vi "BonOMM-SAOMM.vi"() -> ()   [LabVIEW 2019] (continued)
                    n4150 = Concatenate Strings("FAPG.set -> (", w1579, ")") -> (w1577:string)
                    n4151 = call "TERMINAL.vi"("Indicateur Refnum"=w1582, "Terminal Refnum"=w1581, "Indicateur d'état"=w1577) -> ()
                    n4152 = call "SAOMM-SendSET.vi"("PRAMMS-COMM IN"=w1590, "Active Refnum"=w1588, "PrAMS-ACK"=w1587, "Signature"=w1584, "Error IN"=w1589, "MessageType"=w1586, "Active SET"="emtSetFPGACtrl", "Value (little endianed byte array)"=w1583) -> ("PRAMMS-COMM OUT"=w1592:refnum<visa-resource-name>, "Error OUT"=w1591:errorcluster)  [unwired: 4 in, 2 out]
                    n4153 = local write "PrAMS Error"(w1591) -> ()
                    n4154 = local write "PrAMS VRN"(w1592) -> ()
                  }
                  frame True {
                    n4155 = One Button Dialog(message="Impossible de modifier le FPGActrl pendant que la caméra fonctionne") -> ()  [unwired: 1 in, 1 out]
                  }
                }
              }
              event "Binning": Value Change {
                n4156 = event-data() -> ("OldVal"=w1598:u16, "NewVal"=w1597:u16)  [unwired: 1 in, 3 out]
                n4157 = local read "Integrating"() -> (w1595:bool)
                n4158 = local read "Servo"() -> (w1594:bool)
                n4159 = Or(x=w1595, y=w1594) -> (x .or. y?=w1596:bool)
                n4160 = case shown="Faux" w1596 {
                  tunnel: w1598 -> [w1610 _]
                  tunnel: w1597 -> [w1608 _]
                  frame False {
                    w1622 = "cam_Binning "
                    # "Passer dans une astrométrie ?"
                    n4161 = flat-sequence {
                      tunnel: [w1655] -> w1638
                      tunnel: [w1671] -> w1637
                      tunnel: w1638 -> [w1671]
                      tunnel: w1609 -> [w1663]
                      tunnel: w1607 -> [w1662]
                      tunnel: w1606 -> [w1661]
                      tunnel: [w1660] -> w1636
                      tunnel: [w1659] -> w1635
                      tunnel: [w1658] -> w1634
                      tunnel: w1637 -> [w1685]
                      tunnel: [w1682] -> w1605
                      tunnel: w1636 -> [w1682]
                      tunnel: w1635 -> [w1681]
                      tunnel: w1634 -> [w1676]
                      frame #0 {
                        n4162 = Tick Count (ms)() -> (millisecond timer value=w1655:u32)
                      }
                      frame #1 {
                        n4163 = control-ref of="PrAMS-ACK"() -> (w1656:refnum<vi>)
                        n4164 = local read "MessageType"() -> (w1665:cluster{string[], u32[]})
                        n4165 = control-ref of="PrAMS actif"() -> (w1657:refnum<vi>)
                        n4166 = local read "Signature"() -> (w1664:u32)
                        n4167 = local read "PrAMS VRN"() -> (w1670:refnum<visa-resource-name>)
                        n4168 = local read "PrAMS Error"() -> (w1669:errorcluster)
                        n4169 = call "SAOMM-BinningFixer.vi"("PRAMMS-COMM IN"=w1670, "Active Refnum"=w1657, "PrAMS-ACK"=w1656, "Signature"=w1664, "SendSET"=TRUE, "MessageType"=w1665, "Error IN"=w1669, "Binning"=w1663, "NAXIS"=w1661, "ROI Sizes"=w1662) -> ("PRAMMS-COMM OUT"=w1668:refnum<visa-resource-name>, "ScaleFactor"=w1660:dbl, "ROISizesOut"=w1659:T51, "ROIMinMax"=w1658:T52, "Error OUT"=w1667:errorcluster)  [unwired: 1 in]
                        n4170 = local write "PrAMS Error"(w1667) -> ()
                        n4171 = local write "PrAMS VRN"(w1668) -> ()
                      }
                      frame #2 {
                        n4172 = Tick Count (ms)() -> (millisecond timer value=w1684:u32)
                        n4173 = Subtract(x=w1684, y=w1685) -> (x-y=→"SetBinningTime":u32)
                        n4174 = Unbundle(w1681) -> ("ROIXOffset OUT"=w1680:u16, "ROIYOffset OUT"=w1679:u16, "ROIWidth OUT"=w1678:u16, "ROIHeight OUT"=w1677:u16)
                        n4175 = Unbundle(w1676) -> ("ROIXMin"=→"ROIXMin":u16, "ROIYXMax"=→"ROIXMax":u16, "ROIYMin"=→"ROIYMin":u16, "ROIYMax"=→"ROIYMax":u16)
                        n4176 = local write "ROIXOffset"(w1680) -> ()
                        n4177 = local write "ROIYOffset"(w1679) -> ()
                        n4178 = local write "ROIWidth"(w1678) -> ()
                        n4179 = local write "ROIHeight"(w1677) -> ()
                      }
                    }
                    n4180 = local read "Naxis1"() -> (w1599:u16)
                    n4181 = local read "Naxis2"() -> (w1600:u16)
                    n4182 = local read "ROIXOffset"() -> (w1604:u16)
                    n4183 = local read "ROIYOffset"() -> (w1603:u16)
                    n4184 = local read "ROIWidth"() -> (w1602:u16)
                    n4185 = local read "ROIHeight"() -> (w1601:u16)
                    n4186 = Bundle("OldVal"=w1610, "NewVal"=w1608) -> (w1609:cluster{"OldVal":u16, "NewVal":u16})  [unwired: 1 in]
                    n4187 = Bundle("Naxis1"=w1599, "Naxis2"=w1600) -> (w1606:cluster{"Naxis1":u16, "Naxis2":u16})  [unwired: 1 in]
                    n4188 = Bundle("ROIXOffset"=w1604, "ROIYOffset"=w1603, "ROIWidth"=w1602, "ROIHeight"=w1601) -> (w1607:T53)  [unwired: 1 in]
                    n4189 = property on="ImgArray" class="GraphInt (strict)"() -> ("Cursor.Cursor X"=w1633:dbl, "Cursor.Cursor Y"=w1632:dbl)  [unwired: 2 in, 2 out]
                    n4190 = case shown="2" w1608 {
                      tunnel: [TRUE FALSE FALSE FALSE] -> w1614
                      tunnel: [FALSE TRUE FALSE FALSE] -> w1613
                      tunnel: [FALSE FALSE TRUE FALSE] -> w1612
                      tunnel: [FALSE FALSE FALSE TRUE] -> w1611
                      frame 1, Default {
                      }
                      frame 2 {
                      }
                      frame 4 {
                      }
                      frame 5 {
                      }
                    }
                    n4191 = Multiply(x=w1605, y=w1633) -> (x*y=w1631:dbl)
                    n4192 = Multiply(x=w1632, y=w1605) -> (x*y=w1630:dbl)
                    n4193 = Round To Nearest(number=w1631) -> (nearest integer value=w1629:dbl)
                    n4194 = Round To Nearest(number=w1630) -> (nearest integer value=w1628:dbl)
                    n4195 = Current VI's Menubar() -> (w1627:refnum<k9>)
                    n4196 = Concatenate Strings(w1622, "1x1" ("string")) -> (w1623:string)
                    n4197 = Set Menu Item Info(6:w1614, 7:w1623, 11:w1627) -> (3:w1626:refnum<k9>)  [unwired: 4 in, 1 out]
                    n4198 = Concatenate Strings(w1622, "2x2" ("string")) -> (w1617:string)
                    n4199 = Set Menu Item Info(6:w1613, 7:w1617, 11:w1626) -> (3:w1625:refnum<k9>)  [unwired: 4 in, 1 out]
                    n4200 = local write "YReference"(w1628) -> ()
                    n4201 = local write "XReference"(w1629) -> ()
                    n4202 = Concatenate Strings(w1622, "4x4" ("string")) -> (w1616:string)
                    n4203 = Set Menu Item Info(6:w1612, 7:w1616, 11:w1625) -> (3:w1624:refnum<k9>)  [unwired: 4 in, 1 out]
                    n4204 = Concatenate Strings(w1622, "5x5" ("string")) -> (w1615:string)
                    n4205 = property on="ImgArray" class="GraphInt (strict)"("Cursor.Cursor X"=w1629, "Cursor.Cursor Y"=w1628) -> ()  [unwired: 2 in, 2 out]
                    n4206 = Set Menu Item Info(6:w1611, 7:w1615, 11:w1624) -> ()  [unwired: 4 in, 2 out]
                  }
                  frame True {
                  }
                }
              }
              event "EMGain": Value Change {
                n4207 = event-data() -> ("NewVal"=w1689:u16)  [unwired: 1 in, 4 out]
                n4208 = local read "Integrating"() -> (w1687:bool)
                n4209 = local read "Servo"() -> (w1688:bool)
                n4210 = Or(x=w1688, y=w1687) -> (x .or. y?=w1686:bool)
                n4211 = case shown="Faux" w1686 {
                  tunnel: w1689 -> [w1690 _]
                  frame False {
                    n4212 = call-poly "SAOMM-Num2littleEndian.vi"("Number"=w1690) -> ("LiitleEndianedData"=w1691:u8[])  [unwired: 14 in]
                    n4213 = local read "MessageType"() -> (w1694:cluster{string[], u32[]})
                    n4214 = control-ref of="PrAMS-ACK"() -> (w1695:refnum<vi>)
                    n4215 = control-ref of="PrAMS actif"() -> (w1696:refnum<vi>)
                    n4216 = local read "PrAMS VRN"() -> (w1698:refnum<visa-resource-name>)
                    n4217 = local read "PrAMS Error"() -> (w1697:errorcluster)
                    n4218 = local read "Signature"() -> (w1692:u32)
                    n4219 = call "SAOMM-SendSET.vi"("PRAMMS-COMM IN"=w1698, "Active Refnum"=w1696, "PrAMS-ACK"=w1695, "Signature"=w1692, "Error IN"=w1697, "MessageType"=w1694, "Active SET"="emtSetImageEMGain", "Value (little endianed byte array)"=w1691) -> ("PRAMMS-COMM OUT"=w1700:refnum<visa-resource-name>, "Error OUT"=w1699:errorcluster)  [unwired: 4 in, 2 out]
                    n4220 = local write "PrAMS Error"(w1699) -> ()
                    n4221 = local write "PrAMS VRN"(w1700) -> ()
                  }
                  frame True {
                  }
                }
              }
              event "GoCam": Value Change {
                n4222 = event-data() -> ()  [unwired: 1 in, 5 out]
                n4223 = flat-sequence {
                  tunnel: [w1704] -> w1702
                  tunnel: [w1707] -> w1701
                  tunnel: w1702 -> [w1707]
                  tunnel: w1701 -> [w1718]
                  frame #0 {
                    n4224 = local write "GoCam"(FALSE ("GoCam")) -> ()
                    n4225 = Tick Count (ms)() -> (millisecond timer value=w1704:u32)
                  }
                  frame #1 {
                    # "emtStartAcquisition ne prend pas d'arguments"
                    n4226 = local read "MessageType"() -> (w1709:cluster{string[], u32[]})
                    n4227 = control-ref of="PrAMS-ACK"() -> (w1710:refnum<vi>)
                    n4228 = control-ref of="PrAMS actif"() -> (w1711:refnum<vi>)
                    n4229 = local read "PrAMS Error"() -> (w1712:errorcluster)
                    n4230 = local read "PrAMS VRN"() -> (w1713:refnum<visa-resource-name>)
                    n4231 = local read "Signature"() -> (w1705:u32)
                    n4232 = call "SAOMM-SendSET.vi"("PRAMMS-COMM IN"=w1713, "Active Refnum"=w1711, "PrAMS-ACK"=w1710, "Signature"=w1705, "Error IN"=w1712, "MessageType"=w1709, "Active SET"="emtStartAcquisition", "Value (little endianed byte array)"=u8[] []) -> ("PRAMMS-COMM OUT"=w1715:refnum<visa-resource-name>, "Error OUT"=w1714:errorcluster)  [unwired: 4 in, 2 out]
                    n4233 = local write "PrAMS Error"(w1714) -> ()
                    n4234 = local write "PrAMS VRN"(w1715) -> ()
                  }
                  frame #2 {
                    n4235 = Tick Count (ms)() -> (millisecond timer value=w1717:u32)
                    n4236 = Subtract(x=w1717, y=w1718) -> (x-y=→"StartTime":u32)
                  }
                }
              }
              event "StopCam": Value Change {
                n4237 = event-data() -> ()  [unwired: 1 in, 5 out]
                n4238 = flat-sequence {
                  tunnel: [w1722] -> w1720
                  tunnel: [w1725] -> w1719
                  tunnel: w1720 -> [w1725]
                  tunnel: w1719 -> [w1736]
                  frame #0 {
                    n4239 = local write "StopCam"(FALSE ("StopCam")) -> ()
                    n4240 = Tick Count (ms)() -> (millisecond timer value=w1722:u32)
                  }
                  frame #1 {
                    # "emtStartAcquisition ne prend pas d'arguments"
                    n4241 = control-ref of="PrAMS-ACK"() -> (w1728:refnum<vi>)
                    n4242 = local read "PrAMS VRN"() -> (w1731:refnum<visa-resource-name>)
                    n4243 = local read "PrAMS Error"() -> (w1730:errorcluster)
                    n4244 = local read "MessageType"() -> (w1727:cluster{string[], u32[]})
                    n4245 = control-ref of="PrAMS actif"() -> (w1729:refnum<vi>)
                    n4246 = local read "Signature"() -> (w1723:u32)
                    n4247 = call "SAOMM-SendSET.vi"("PRAMMS-COMM IN"=w1731, "Active Refnum"=w1729, "PrAMS-ACK"=w1728, "Signature"=w1723, "Error IN"=w1730, "MessageType"=w1727, "Active SET"="emtStopAcquisition", "Value (little endianed byte array)"=u8[] []) -> ("PRAMMS-COMM OUT"=w1733:refnum<visa-resource-name>, "Error OUT"=w1732:errorcluster)  [unwired: 4 in, 2 out]
                    n4248 = local write "PrAMS Error"(w1732) -> ()
                    n4249 = local write "PrAMS VRN"(w1733) -> ()
                  }
                  frame #2 {
                    n4250 = Tick Count (ms)() -> (millisecond timer value=w1735:u32)
                    n4251 = Subtract(x=w1735, y=w1736) -> (x-y=→"StopTime":u32)
                  }
                }
              }
              event "ROIsurface": Value Change {
                n4252 = event-data() -> ()  [unwired: 1 in, 5 out]
                n4253 = local read "Mode"() -> (w1739:u16)
                n4254 = local read "Servo"() -> (w1740:bool)
                n4255 = Equal?(x=w1739, y=u16 2) -> (x = y?=w1737:bool)
                n4256 = And(x=w1740, y=w1737) -> (x .and. y?=w1741:bool)
                n4257 = case shown="Faux" w1741 {
                  frame False {
                    w1753 = 0.0 ("y")
                    # "Pour l'instant, on met le pixel de référence au centre de la ROI"
                    # "Est-ce que le binning ne devrait pas apparaître ici ?!?"
                    n4258 = control-ref of="PrAMS-ACK"() -> (w1758:refnum<vi>)
                    n4259 = local read "MessageType"() -> (w1757:cluster{string[], u32[]})
                    n4260 = control-ref of="PrAMS actif"() -> (w1759:refnum<vi>)
                    n4261 = local read "Signature"() -> (w1763:u32)
                    n4262 = local read "PrAMS VRN"() -> (w1767:refnum<visa-resource-name>)
                    n4263 = local read "PrAMS Error"() -> (w1760:errorcluster)
                    n4264 = local read "ROISizes"() -> (w1773:u16[])
                    n4265 = call-poly "SAOMM-Num2littleEndian.vi"("Number"=w1753) -> ("LiitleEndianedData"=w1755:u8[])  [unwired: 14 in]
                    n4266 = call-poly "SAOMM-Num2littleEndian.vi"("Number"=w1753) -> ("LiitleEndianedData"=w1754:u8[])  [unwired: 14 in]
                    n4267 = Index Array(array=w1773, index="ROIsurface") -> (element=w1745:u16)
                    n4268 = call "SAOMM-SendSET.vi"("PRAMMS-COMM IN"=w1767, "Active Refnum"=w1759, "PrAMS-ACK"=w1758, "Signature"=w1763, "Error IN"=w1760, "MessageType"=w1757, "Active SET"="emtSetROIXReferencePoint", "Value (little endianed byte array)"=w1755) -> ("PRAMMS-COMM OUT"=w1769:refnum<visa-resource-name>, "Error OUT"=w1768:errorcluster)  [unwired: 4 in, 2 out]
                    n4269 = local write "ROIWidth"(w1745) -> ()
                    n4270 = local write "ROIHeight"(w1745) -> ()
                    n4271 = call-poly "SAOMM-Num2littleEndian.vi"("Number"=w1745) -> ("LiitleEndianedData"=w1777:u8[])  [unwired: 14 in]
                    n4272 = call "SAOMM-SendSET.vi"("PRAMMS-COMM IN"=w1769, "Active Refnum"=w1759, "PrAMS-ACK"=w1758, "Signature"=w1763, "Error IN"=w1768, "MessageType"=w1757, "Active SET"="emtSetROIYReferencePoint", "Value (little endianed byte array)"=w1754) -> ("PRAMMS-COMM OUT"=w1766:refnum<visa-resource-name>)  [unwired: 4 in, 3 out]
                    n4273 = call "SAOMM-SendSET.vi"("PRAMMS-COMM IN"=w1766, "Active Refnum"=w1759, "PrAMS-ACK"=w1758, "Signature"=w1763, "MessageType"=w1757, "Active SET"="emtSetROIWidth", "Value (little endianed byte array)"=w1777) -> ("PRAMMS-COMM OUT"=w1776:refnum<visa-resource-name>, "Error OUT"=w1775:errorcluster)  [unwired: 5 in, 2 out]
                    n4274 = call "SAOMM-SendSET.vi"("PRAMMS-COMM IN"=w1776, "Active Refnum"=w1759, "PrAMS-ACK"=w1758, "Signature"=w1763, "Error IN"=w1775, "MessageType"=w1757, "Active SET"="emtSetROIHeight", "Value (little endianed byte array)"=w1777) -> ("PRAMMS-COMM OUT"=w1765:refnum<visa-resource-name>, "Error OUT"=w1762:errorcluster)  [unwired: 4 in, 2 out]
                    n4275 = To Double Precision Float(number=w1745) -> (double precision float=w1746:dbl)
                    n4276 = To Double Precision Float(number=w1745) -> (double precision float=w1744:dbl)
                    n4277 = expression code="x/2.0"(w1746) -> (w1743:dbl)
                    n4278 = expression code="x/2.0"(w1744) -> (w1742:dbl)
                    n4279 = local write "XROIRef"(w1743) -> ()
                    n4280 = local write "YROIRef"(w1742) -> ()
                    n4281 = call-poly "SAOMM-Num2littleEndian.vi"("Number"=w1743) -> ("LiitleEndianedData"=w1748:u8[])  [unwired: 14 in]
                    n4282 = call-poly "SAOMM-Num2littleEndian.vi"("Number"=w1742) -> ("LiitleEndianedData"=w1747:u8[])  [unwired: 14 in]
                    n4283 = call "SAOMM-SendSET.vi"("PRAMMS-COMM IN"=w1765, "Active Refnum"=w1759, "PrAMS-ACK"=w1758, "Signature"=w1763, "Error IN"=w1762, "MessageType"=w1757, "Active SET"="emtSetROIXReferencePoint", "Value (little endianed byte array)"=w1748) -> ("PRAMMS-COMM OUT"=w1770:refnum<visa-resource-name>, "Error OUT"=w1771:errorcluster)  [unwired: 4 in, 2 out]
                    n4284 = call "SAOMM-SendSET.vi"("PRAMMS-COMM IN"=w1770, "Active Refnum"=w1759, "PrAMS-ACK"=w1758, "Signature"=w1763, "Error IN"=w1771, "MessageType"=w1757, "Active SET"="emtSetROIYReferencePoint", "Value (little endianed byte array)"=w1747) -> ("PRAMMS-COMM OUT"=w1764:refnum<visa-resource-name>, "Error OUT"=w1761:errorcluster)  [unwired: 4 in, 2 out]
                    n4285 = local write "PrAMS Error"(w1761) -> ()
                    n4286 = local write "PrAMS VRN"(w1764) -> ()
                  }
                  frame True {
                  }
                }
              }
              event "UpdateROI": Value Change {
                n4287 = event-data() -> ()  [unwired: 1 in, 5 out]
                n4288 = local read "Servo"() -> (w1778:bool)
                n4289 = case shown="Faux" w1778 {
                  frame False {
                    n4290 = flat-sequence {
                      tunnel: [w1782] -> w1780
                      tunnel: [w1817] -> w1779
                      tunnel: w1780 -> [w1817]
                      tunnel: w1779 -> [w1820]
                      frame #0 {
                        n4291 = local write "UpdateROI"(FALSE) -> ()
                        n4292 = Tick Count (ms)() -> (millisecond timer value=w1782:u32)
                      }
                      frame #1 {
                        n4293 = local read "Binning"() -> (w1808:u16)
                        n4294 = local read "ROIWidth"() -> (w1799:u16)
                        n4295 = local read "ROIHeight"() -> (w1800:u16)
                        n4296 = local read "Naxis1"() -> (w1806:u16)
                        n4297 = local read "Naxis2"() -> (w1805:u16)
                        n4298 = local read "ROIXOffset"() -> (w1801:u16)
                        n4299 = local read "ROIYOffset"() -> (w1802:u16)
                        n4300 = local read "XROIRef"() -> (w1797:dbl)
                        n4301 = local read "YROIRef"() -> (w1796:dbl)
                        n4302 = Bundle("XROIRef"=w1797, "YROIRef"=w1796) -> (w1798:cluster{"XROIRef":dbl, "YROIRef":dbl})  [unwired: 1 in]
                        n4303 = Bundle("Naxis1"=w1806, "Naxis2"=w1805) -> (w1807:cluster{"Naxis1":u16, "Naxis2":u16})  [unwired: 1 in]
                        n4304 = Bundle("ROIWidth"=w1799, "ROIHeight"=w1800) -> (w1804:cluster{"ROIWidth":u16, "ROIHeight":u16})  [unwired: 1 in]
                        n4305 = Bundle("ROIXOffset"=w1801, "ROIYOffset"=w1802) -> (w1803:cluster{"ROIXOffset":u16, "ROIYOffset":u16})  [unwired: 1 in]
                        n4306 = call "SAOMM-ROI_Fixer.vi"("Binning"=w1808, "Use Offset?"=TRUE, "naxis"=w1807, "ROI"=w1804, "Offset"=w1803, "Reference Pixel"=w1798) -> ("FixedOffset"=w1785:cluster{"ROIXOffset":u16, "ROIYOffset":u16}, "FixedPixel"=w1783:cluster{"PixelX":dbl, "PixelY":dbl})  [unwired: 6 in, 2 out]
                        n4307 = Unbundle By Name(w1785) -> ("ROIXOffset"=w1795:u16, "ROIYOffset"=w1794:u16)
                        n4308 = control-ref of="PrAMS-ACK"() -> (w1811:refnum<vi>)
                        n4309 = local read "MessageType"() -> (w1810:cluster{string[], u32[]})
                        n4310 = control-ref of="PrAMS actif"() -> (w1816:refnum<vi>)
                        n4311 = local read "PrAMS VRN"() -> (w1815:refnum<visa-resource-name>)
                        n4312 = local read "PrAMS Error"() -> (w1814:errorcluster)
                        n4313 = Unbundle By Name(w1783) -> ("PixelX"=w1786:dbl, "PixelY"=w1789:dbl)
                        n4314 = Bundle("ROIYOffset"=w1794, "ROIXOffset"=w1795) -> (w1784:cluster{"ROIYOffset":u16, "ROIXOffset":u16})  [unwired: 1 in]
                        n4315 = local write "XReference"(w1786) -> ()
                        n4316 = local write "YReference"(w1789) -> ()
                        n4317 = To Double Precision Float(number=w1795) -> (double precision float=w1788:dbl)
                        n4318 = To Double Precision Float(number=w1794) -> (double precision float=w1787:dbl)
                        n4319 = call "SAOMM-UpdateROI.vi"("PRAMMS-COMM IN"=w1815, "Active Refnum"=w1816, "PrAMS-ACK"=w1811, "MessageType"=w1810, "Error IN"=w1814, "Position"=w1784) -> ("PRAMMS-COMM OUT"=w1813:refnum<visa-resource-name>, "Error OUT"=w1812:errorcluster)  [unwired: 7 in, 1 out]
                        n4320 = property on="ImgArray" class="GraphInt (strict)"() -> ("Cursor.Cursor Position"=w1793:T45)  [unwired: 2 in, 2 out]
                        n4321 = local write "PrAMS Error"(w1812) -> ()
                        n4322 = local write "PrAMS VRN"(w1813) -> ()
                        n4323 = Add(x=w1787, y=w1786) -> (x+y=w1790:dbl)
                        n4324 = Add(x=w1788, y=w1789) -> (x+y=w1791:dbl)
                        n4325 = Bundle(cluster=w1793, "Cursor X"=w1790, "Cursor Y"=w1791) -> (w1792:T45)
                        n4326 = property on="ImgArray" class="GraphInt (strict)"("Cursor.Cursor Position"=w1792) -> ()  [unwired: 2 in, 2 out]
                      }
                      frame #2 {
                        n4327 = Tick Count (ms)() -> (millisecond timer value=w1819:u32)
                        n4328 = Subtract(x=w1819, y=w1820) -> (x-y=→"SetROITime":u32)
                      }
                    }
                  }
                  frame True {
                    n4329 = local read "FIFO d'erreur"() -> (w1822:T7)
                    n4330 = call "Error_Format.vi"("FIFO IN"=w1822, "Source"="PrAMS", "Comment"="Impossible de modifier les paramères de la ROI pendant l'asserviseement.") -> ("FIFO OUT"=w1823:T7)  [unwired: 14 in, 2 out]
                    n4331 = local write "FIFO d'erreur"(w1823) -> ()
                  }
                }
              }
              event "Milieu": Value Change {
                # "Calcul les paramètres du milieu"
                n4332 = event-data() -> ()  [unwired: 1 in, 5 out]
                n4333 = local read "Binning"() -> (w1832:u16)
                n4334 = local read "ROIWidth"() -> (w1836:u16)
                n4335 = local read "ROIHeight"() -> (w1835:u16)
                n4336 = local read "Naxis1"() -> (w1833:u16)
                n4337 = local read "Naxis2"() -> (w1834:u16)
                n4338 = formula code="Xoff=((nax1/bin)-ROIw)/2;\nYoff=((nax2/bin)-ROIh)/2;"("bin"=w1832, "nax1"=w1833, "nax2"=w1834, "ROIw"=w1836, "ROIh"=w1835) -> ("Xoff"=w1831:dbl, "Yoff"=w1829:dbl)
                n4339 = local read "XROIRef"() -> (w1838:dbl)
                n4340 = local read "YROIRef"() -> (w1837:dbl)
                n4341 = local write "Milieu"(FALSE ("Use Offset?")) -> ()
                n4342 = Bundle("XROIRef"=w1838, "YROIRef"=w1837) -> (w1850:cluster{"XROIRef":dbl, "YROIRef":dbl})  [unwired: 1 in]
                n4343 = To Unsigned Word Integer(number=w1831) -> (unsigned 16bit integer=w1830:u16)
                n4344 = To Unsigned Word Integer(number=w1829) -> (unsigned 16bit integer=w1828:u16)
                n4345 = Bundle("Naxis1"=w1833, "Naxis2"=w1834) -> (w1853:cluster{"Naxis1":u16, "Naxis2":u16})  [unwired: 1 in]
                n4346 = Bundle("ROIWidth"=w1836, "ROIHeight"=w1835) -> (w1852:cluster{"ROIWidth":u16, "ROIHeight":u16})  [unwired: 1 in]
                n4347 = local write "ROIXOffset"(w1830) -> ()
                n4348 = local write "ROIYOffset"(w1828) -> ()
                n4349 = Bundle(w1830, w1828) -> (w1851:cluster{u16, u16})  [unwired: 1 in]
                n4350 = call "SAOMM-ROI_Fixer.vi"("Binning"=w1832, "Use Offset?"=TRUE, "naxis"=w1853, "ROI"=w1852, "Offset"=w1851, "Reference Pixel"=w1850) -> ("FixedOffset"=w1841:cluster{"ROIXOffset":u16, "ROIYOffset":u16}, "FixedPixel"=w1839:cluster{"PixelX":dbl, "PixelY":dbl})  [unwired: 6 in, 2 out]
                n4351 = control-ref of="PrAMS-ACK"() -> (w1856:refnum<vi>)
                n4352 = local read "MessageType"() -> (w1855:cluster{string[], u32[]})
                n4353 = control-ref of="PrAMS actif"() -> (w1861:refnum<vi>)
                n4354 = local read "PrAMS VRN"() -> (w1860:refnum<visa-resource-name>)
                n4355 = local read "PrAMS Error"() -> (w1859:errorcluster)
                n4356 = Unbundle By Name(w1841) -> ("ROIXOffset"=w1849:u16, "ROIYOffset"=w1848:u16)
                n4357 = Unbundle By Name(w1839) -> ("PixelX"=w1842:dbl, "PixelY"=w1845:dbl)
                n4358 = To Double Precision Float(number=w1849) -> (double precision float=w1844:dbl)
                n4359 = To Double Precision Float(number=w1848) -> (double precision float=w1843:dbl)
                n4360 = Bundle("ROIYOffset"=w1848, "ROIXOffset"=w1849) -> (w1840:cluster{"ROIYOffset":u16, "ROIXOffset":u16})  [unwired: 1 in]
                n4361 = property on="ImgArray" class="GraphInt (strict)"() -> ("Cursor.Cursor Position"=w1847:T45)  [unwired: 2 in, 2 out]
                n4362 = Add(x=w1843, y=w1842) -> (x+y=w1827:dbl)
                n4363 = Add(x=w1844, y=w1845) -> (x+y=w1826:dbl)
                n4364 = call "SAOMM-UpdateROI.vi"("PRAMMS-COMM IN"=w1860, "Active Refnum"=w1861, "PrAMS-ACK"=w1856, "MessageType"=w1855, "Error IN"=w1859, "Position"=w1840) -> ("PRAMMS-COMM OUT"=w1858:refnum<visa-resource-name>, "Error OUT"=w1857:errorcluster)  [unwired: 7 in, 1 out]
                n4365 = local write "PrAMS Error"(w1857) -> ()
                n4366 = local write "XReference"(w1827) -> ()
                n4367 = local write "PrAMS VRN"(w1858) -> ()
                n4368 = local write "YReference"(w1826) -> ()
                n4369 = Bundle(cluster=w1847, "Cursor X"=w1827, "Cursor Y"=w1826) -> (w1846:T45)
                n4370 = property on="ImgArray" class="GraphInt (strict)"("Cursor.Cursor Position"=w1846) -> ()  [unwired: 2 in, 2 out]
              }
              event "FalconProcessed": Value Change {
                n4371 = event-data() -> ()  [unwired: 1 in, 5 out]
                n4372 = case shown="Vrai" "FalconProcessed" {
                  frame False {
                  }
                  frame True {
                    n4373 = local write "FalconProcessed"(FALSE ("FalconProcessed")) -> ()
                    n4374 = local read "Nb_FalconProc_demandé"() -> (w1863:u32)
                    n4375 = local read "MessageType"() -> (w1869:cluster{string[], u32[]})
                    n4376 = control-ref of="PrAMS actif"() -> (w1870:refnum<vi>)
                    n4377 = local read "PrAMS VRN"() -> (w1866:refnum<visa-resource-name>)
                    n4378 = local read "PrAMS Error"() -> (w1871:errorcluster)
                    n4379 = Increment(x=w1863) -> (x+1=→"Nb_FalconProc_demandé":u32)
                    n4380 = local read "Signature"() -> (w1867:u32)
                    n4381 = call "SAOMM-SendGET.vi"("PRAMMS-COMM IN"=w1866, "Bool Refnum"=w1870, "MessageType"=w1869, "Signature"=w1867, "Error IN"=w1871, "Active GET"="emtGetProcessedFalconImage" ("Active SET")) -> ("PRAMMS-COMM OUT"=w1865:refnum<visa-resource-name>, "Error OUT"=w1872:errorcluster)  [unwired: 8 in]
                    n4382 = local write "PrAMS VRN"(w1865) -> ()
                    n4383 = local write "PrAMS Error"(w1872) -> ()
                  }
                }
              }
              event "QueryServoLevel": Value Change {
                n4384 = event-data() -> ("NewVal"=w1874:bool)  [unwired: 1 in, 4 out]
                n4385 = case shown="Vrai" w1874 {
                  frame False {
                  }
                  frame True {
                    n4386 = local read "MessageType"() -> (w1880:cluster{string[], u32[]})
                    n4387 = control-ref of="PrAMS actif"() -> (w1879:refnum<vi>)
                    n4388 = local read "PrAMS VRN"() -> (w1877:refnum<visa-resource-name>)
                    n4389 = local read "PrAMS Error"() -> (w1878:errorcluster)
                    n4390 = local read "Signature"() -> (w1876:u32)
                    n4391 = call "SAOMM-SendGET.vi"("PRAMMS-COMM IN"=w1877, "Bool Refnum"=w1879, "MessageType"=w1880, "Signature"=w1876, "Error IN"=w1878, "Active GET"="emtGetTelescopeServoLevel" ("Active SET")) -> ("PRAMMS-COMM OUT"=w1882:refnum<visa-resource-name>, "Error OUT"=w1883:errorcluster)  [unwired: 8 in]
                    n4392 = local write "PrAMS VRN"(w1882) -> ()
                    n4393 = local write "PrAMS Error"(w1883) -> ()
                  }
                }
                n4394 = local write "QueryServoLevel"(FALSE ("QueryServoLevel")) -> ()
              }
              event "GetOptimal": Value Change {
                # "[quote=\"TELOPS\"] Ne sera pas implémenter par manque de temps ... [/quote]"
                n4395 = event-data() -> ()  [unwired: 1 in, 5 out]
                n4396 = flat-sequence {
                  tunnel: [w1887] -> w1885
                  tunnel: [w1889] -> w1884
                  tunnel: w1885 -> [w1889]
                  tunnel: w1884 -> [w1897]
                  frame #0 {
                    n4397 = local write "GetOptimal"(FALSE ("GetOptimal")) -> ()
                    n4398 = Tick Count (ms)() -> (millisecond timer value=w1887:u32)
                  }
                  frame #1 {
                    n4399 = local read "MessageType"() -> (w1891:cluster{string[], u32[]})
                    n4400 = control-ref of="PrAMS actif"() -> (w1892:refnum<vi>)
                    n4401 = local read "PrAMS Error"() -> (w1893:errorcluster)
                    n4402 = local read "PrAMS VRN"() -> (w1894:refnum<visa-resource-name>)
                    n4403 = local read "Signature"() -> (w1888:u32)
                    n4404 = call "SAOMM-SendGET.vi"("PRAMMS-COMM IN"=w1894, "Bool Refnum"=w1892, "MessageType"=w1891, "Signature"=w1888, "Error IN"=w1893, "Active GET"="emtGetOptimalExposureTime" ("Active SET")) -> ("PRAMMS-COMM OUT"=w1896:refnum<visa-resource-name>, "Error OUT"=w1895:errorcluster)  [unwired: 8 in]
                    n4405 = local write "PrAMS Error"(w1895) -> ()
                    n4406 = local write "PrAMS VRN"(w1896) -> ()
                  }
                  frame #2 {
                    "GetOptimalTime" <- w1897
                  }
                }
              }
              event "AutoCentroid": Value Change {
                # "À vérifier ...\nSemble ok : 2013-09-20"
                n4407 = event-data() -> ()  [unwired: 1 in, 5 out]
                n4408 = local write "AutoCentroid"(FALSE ("AutoCentroid")) -> ()
                n4409 = local read "XCentroid"() -> (w1919:dbl)
                n4410 = local read "YCentroid"() -> (w1920:dbl)
                n4411 = local read "XROIRef"() -> (w1903:dbl)
                n4412 = local read "YROIRef"() -> (w1902:dbl)
                n4413 = Subtract(x=w1919, y=w1903) -> (x-y=w1939:dbl)
                n4414 = Subtract(x=w1920, y=w1902) -> (x-y=w1938:dbl)
                n4415 = Round To Nearest(number=w1939) -> (nearest integer value=w1937:dbl)
                n4416 = Round To Nearest(number=w1938) -> (nearest integer value=w1936:dbl)
                n4417 = To Unsigned Word Integer(number=w1937) -> (unsigned 16bit integer=w1925:u16)
                n4418 = To Unsigned Word Integer(number=w1936) -> (unsigned 16bit integer=w1924:u16)
                n4419 = local read "Binning"() -> (w1934:u16)
                n4420 = local read "ROIWidth"() -> (w1927:u16)
                n4421 = local read "ROIHeight"() -> (w1928:u16)
                n4422 = local read "Naxis1"() -> (w1932:u16)
                n4423 = local read "Naxis2"() -> (w1931:u16)
                n4424 = local read "XROIRef"() -> (w1922:dbl)
                n4425 = local read "YROIRef"() -> (w1921:dbl)
                n4426 = Bundle("XROIRef"=w1922, "YROIRef"=w1921) -> (w1926:cluster{"XROIRef":dbl, "YROIRef":dbl})  [unwired: 1 in]
                n4427 = Bundle("Naxis1"=w1932, "Naxis2"=w1931) -> (w1933:cluster{"Naxis1":u16, "Naxis2":u16})  [unwired: 1 in]
                n4428 = Bundle("ROIWidth"=w1927, "ROIHeight"=w1928) -> (w1930:cluster{"ROIWidth":u16, "ROIHeight":u16})  [unwired: 1 in]
                n4429 = Bundle(w1925, w1924) -> (w1929:cluster{u16, u16})  [unwired: 1 in]
                n4430 = call "SAOMM-ROI_Fixer.vi"("Binning"=w1934, "Use Offset?"=TRUE, "naxis"=w1933, "ROI"=w1930, "Offset"=w1929, "Reference Pixel"=w1926) -> ("FixedOffset"=w1901:cluster{"ROIXOffset":u16, "ROIYOffset":u16}, "FixedPixel"=w1923:cluster{"PixelX":dbl, "PixelY":dbl})  [unwired: 6 in, 2 out]
                n4431 = Unbundle By Name(w1901) -> ("ROIXOffset"=w1898:u16, "ROIYOffset"=w1899:u16)
                n4432 = Unbundle By Name(w1923) -> ("PixelX"=w1911:dbl, "PixelY"=w1908:dbl)
                n4433 = control-ref of="PrAMS-ACK"() -> (w1913:refnum<vi>)
                n4434 = local read "MessageType"() -> (w1912:cluster{string[], u32[]})
                n4435 = Bundle("ROIYOffset"=w1899, "ROIXOffset"=w1898) -> (w1900:cluster{"ROIYOffset":u16, "ROIXOffset":u16})  [unwired: 1 in]
                n4436 = control-ref of="PrAMS actif"() -> (w1918:refnum<vi>)
                n4437 = local write "XReference"(w1911) -> ()
                n4438 = local write "YReference"(w1908) -> ()
                n4439 = local read "PrAMS VRN"() -> (w1917:refnum<visa-resource-name>)
                n4440 = local read "PrAMS Error"() -> (w1916:errorcluster)
                n4441 = property on="ImgArray" class="GraphInt (strict)"() -> ("Cursor.Cursor Position"=w1904:T45)  [unwired: 2 in, 2 out]
                n4442 = To Double Precision Float(number=w1898) -> (double precision float=w1909:dbl)
                n4443 = To Double Precision Float(number=w1899) -> (double precision float=w1910:dbl)
                n4444 = Add(x=w1910, y=w1911) -> (x+y=w1907:dbl)
                n4445 = Add(x=w1909, y=w1908) -> (x+y=w1906:dbl)
                n4446 = call "SAOMM-UpdateROI.vi"("PRAMMS-COMM IN"=w1917, "Active Refnum"=w1918, "PrAMS-ACK"=w1913, "MessageType"=w1912, "Error IN"=w1916, "Position"=w1900) -> ("PRAMMS-COMM OUT"=w1915:refnum<visa-resource-name>, "Error OUT"=w1914:errorcluster)  [unwired: 7 in, 1 out]
                n4447 = Bundle(cluster=w1904, "Cursor X"=w1907, "Cursor Y"=w1906) -> (w1905:T45)
                n4448 = local write "PrAMS Error"(w1914) -> ()
                n4449 = local write "PrAMS VRN"(w1915) -> ()
                n4450 = property on="ImgArray" class="GraphInt (strict)"("Cursor.Cursor Position"=w1905) -> ()  [unwired: 2 in, 2 out]
              }
              event "StartServo": Value Change {
                # "Permet l'annulation des\ncommandes de guidage."
                n4451 = event-data() -> ()  [unwired: 1 in, 5 out]
                n4452 = local write "StartServo"(FALSE ("StartServo")) -> ()
                n4453 = local write "GuidingCancel"(FALSE ("GuidingCancel")) -> ()
                n4454 = case shown="4" "Mode" {
                  tunnel: "Mode" -> [_ w1948 _]
                  frame 0, Default {
                    # "Ici, ce sera le mode \"calibration\" ..."
                  }
                  frame 1..3 {
                    # "Pour lancer le guidage traditionnel, il suffit de\nmettre l'indicateur d'activation à \"vrai\" ... on en\nprofite aussi pour remettre le compteur à zéro."
                    n4455 = flat-sequence {
                      tunnel: w1948 -> [w1952]
                      tunnel: [w1952] -> w1947
                      tunnel: [w1950] -> w1944
                      tunnel: w1947 -> [w1968]
                      tunnel: [w1968] -> w1946
                      tunnel: w1944 -> [w1967]
                      tunnel: w1946 -> [w1979]
                      tunnel: [w1979] -> w1945
                      tunnel: w1945 -> [w2017]
                      frame #0 {
                        w1955 = T17."Disabled and Grayed Out" ("Disabled")
                        w1957 = T17."Disabled" ("Disabled")
                        # "Si le mode est calibration\nC'est qu'on ajuste la collimation"
                        # "Lors de offset, un fichier sera créer à chaque fois :("
                        n4456 = local read "LoggingTimeStamp"() -> (→"GraphTimeStamp":dbl)
                        n4457 = Get Date/Time In Seconds() -> (seconds since 1Jan1904=w1961:timestamp)
                        n4458 = local write "Guidage en cour"(TRUE ("Guidage en cour")) -> ()
                        n4459 = To Double Precision Float(number=w1961) -> (double precision float=w1962:dbl)
                        n4460 = call "GetPathFromTimeStamp.vi"("UTC Time"=TRUE, "LocalTimeStamp"=w1962, "Changement de date à midi ?"=TRUE) -> ("Time String"=w1959:string)  [unwired: 11 in, 1 out]
                        n4461 = Concatenate Strings(w1959, ".gud") -> (→"TrackLogFilename":string)
                        n4462 = property on="StopCam" class="Bool (strict)"("DisabledEnum"=w1955) -> ()  [unwired: 2 in, 2 out]
                        n4463 = property on="StartServo" class="Bool (strict)"("DisabledEnum"=w1955) -> ()  [unwired: 2 in, 2 out]
                        n4464 = property on="AutoCentroid" class="Bool (strict)"("DisabledEnum"=w1955) -> ()  [unwired: 2 in, 2 out]
                        n4465 = property on="Mode" class="MDér (strict)"("DisabledEnum"=w1957) -> ()  [unwired: 2 in, 2 out]
                        n4466 = property on="XReference" class="NumNb (strict)"("DisabledEnum"=w1957) -> ()  [unwired: 2 in, 2 out]
                        n4467 = local write "Flux Min"(inf ("Flux Min")) -> ()
                        n4468 = local write "Flux Max"(0.0 ("Flux Max")) -> ()
                        n4469 = Equal?(x=u16 3, y=w1952) -> (x = y?=w1953:bool)
                        n4470 = property on="Milieu" class="Bool (strict)"("DisabledEnum"=w1955) -> ()  [unwired: 2 in, 2 out]
                        n4471 = property on="GoCam" class="Bool (strict)"("DisabledEnum"=w1955) -> ()  [unwired: 2 in, 2 out]
                        n4472 = property on="GetOptimal" class="Bool (strict)"("DisabledEnum"=w1955) -> ()  [unwired: 2 in, 2 out]
                        n4473 = property on="YReference" class="NumNb (strict)"("DisabledEnum"=w1957) -> ()  [unwired: 2 in, 2 out]
                        n4474 = property on="exptime" class="NumNb (strict)"("DisabledEnum"=w1957) -> ()  [unwired: 2 in, 2 out]
                        n4475 = Select(t=u16 1, s=w1953, f=w1952) -> (s? t:f=w1950:u16)
                      }
                      frame #1 {
                        n4476 = control-ref of="PrAMS-ACK"() -> (w1973:refnum<vi>)
                        n4477 = control-ref of="PrAMS actif"() -> (w1974:refnum<vi>)
                        n4478 = local read "PrAMS VRN"() -> (w1976:refnum<visa-resource-name>)
                        n4479 = local read "PrAMS Error"() -> (w1975:errorcluster)
                        n4480 = local read "MessageType"() -> (w1972:cluster{string[], u32[]})
                        n4481 = local read "Signature"() -> (w1969:u32)
                        n4482 = call-poly "SAOMM-Num2littleEndian.vi"("Number"=w1967) -> ("LiitleEndianedData"=w1970:u8[])  [unwired: 14 in]
                        n4483 = call "SAOMM-SendSET.vi"("PRAMMS-COMM IN"=w1976, "Active Refnum"=w1974, "PrAMS-ACK"=w1973, "Signature"=w1969, "Error IN"=w1975, "MessageType"=w1972, "Active SET"="emtSetTelescopeServoLevel", "Value (little endianed byte array)"=w1970) -> ("PRAMMS-COMM OUT"=w1978:refnum<visa-resource-name>, "Error OUT"=w1977:errorcluster)  [unwired: 4 in, 2 out]
                        n4484 = local write "PrAMS Error"(w1977) -> ()
                        n4485 = local write "PrAMS VRN"(w1978) -> ()
                      }
                      frame #2 {
                        n4486 = case shown="0" w1979 {
                          frame Default {
                          }
                          frame 0 {
                            w1980 = 1.0
                            n4487 = control-ref of="TCS actif"() -> (w1986:refnum<vi>)
                            n4488 = local read "TCS VRN"() -> (w1983:refnum<visa-resource-name>)
                            n4489 = Build Array(w1980) -> (w1984:dbl[])
                            n4490 = expression code="1000/x"(w1980) -> (w1981:dbl)
                            n4491 = call "EXCOM-CMD.vi"("VRN IN"=w1983, "Bool Refnum"=w1986, "Commande #"=15, "Args"=w1984) -> ("VRN OUT"=w1982:refnum<visa-resource-name>)  [unwired: 9 in, 2 out]
                            n4492 = local write "CorrID"(u64 0 ("CorrID")) -> ()
                            n4493 = local write "Servo"(TRUE ("Servo")) -> ()
                            n4494 = local write "TCS VRN"(w1982) -> ()
                            n4495 = local write "RateDEC"(w1981) -> ()
                            n4496 = local write "RateRA"(w1981) -> ()
                          }
                          frame 1 {
                            w1990 = 1.0
                            # "Dans le cas 1, on fonctionne aussi en guidage\ntraditionnel avec un GuiderRate de 1\"/s"
                            n4497 = control-ref of="TCS actif"() -> (w1996:refnum<vi>)
                            n4498 = local read "TCS VRN"() -> (w1993:refnum<visa-resource-name>)
                            n4499 = Build Array(w1990) -> (w1994:dbl[])
                            n4500 = expression code="1000/x"(w1990) -> (w1991:dbl)
                            n4501 = call "EXCOM-CMD.vi"("VRN IN"=w1993, "Bool Refnum"=w1996, "Commande #"=15, "Args"=w1994) -> ("VRN OUT"=w1992:refnum<visa-resource-name>)  [unwired: 9 in, 2 out]
                            n4502 = local write "CorrID"(u64 0 ("CorrID")) -> ()
                            n4503 = local write "TCS VRN"(w1992) -> ()
                            n4504 = local write "RateDEC"(w1991) -> ()
                            n4505 = local write "RateRA"(w1991) -> ()
                          }
                          frame 2 {
                            # "Dans le cas \"2\", on doit modifier la vitesse de guidage\npour l'ajuster au temps d'exposition de la falcon ..."
                            n4506 = local read "exptime"() -> (w2009:dbl)
                            n4507 = Greater?(x=w2009, y=1.25) -> (0:w2007:bool)
                            n4508 = case shown="Vrai" w2007 {
                              frame False {
                              }
                              frame True {
                                n4509 = One Button Dialog(message="Il est fortement conseillé de ne pas utiliser un temps de pose\nde plus de 1.25 secondes pour l'asservissement actif.\n\nAu delà de 3 secondes, le système se comportera très mal.\n\nAssurez-vous que c'est bien ce que vous voulez faire, dans\nle cas contraire, utiliser plutôt le guidage traditionnel." ("Active SET"), button name ("OK")="J'ai lu le message, merci.") -> ()  [unwired: 1 out]
                              }
                            }
                            n4510 = formula code="GuideRate = 0.1288/(2*exptime);\nMillisecondRate=1000/GuideRate;"("exptime"=w2009) -> ("GuideRate"=w2000:dbl, "MillisecondRate"=w1997:dbl)
                            n4511 = In Range and Coerce(upper limit=1.0, x=w2000, lower limit=0.05) -> (coerced(x)=w2001:dbl)  [unwired: 1 out]
                            n4512 = control-ref of="TCS actif"() -> (w2006:refnum<vi>)
                            n4513 = local read "TCS VRN"() -> (w2003:refnum<visa-resource-name>)
                            n4514 = Build Array(w2001) -> (w2004:dbl[])
                            n4515 = call "EXCOM-CMD.vi"("VRN IN"=w2003, "Bool Refnum"=w2006, "Commande #"=15, "Args"=w2004) -> ("VRN OUT"=w2002:refnum<visa-resource-name>)  [unwired: 9 in, 2 out]
                            n4516 = local write "RateDEC"(w1997) -> ()
                            n4517 = local write "TCS VRN"(w2002) -> ()
                            n4518 = local write "RateRA"(w1997) -> ()
                          }
                          frame 3 {
                            n4519 = local write "CorrID"(u64 18446744073709551615 ("CorrID")) -> ()
                          }
                        }
                      }
                      frame #3 {
                        n4520 = local read "XReference"() -> (w2035:dbl)
                        n4521 = local read "YReference"() -> (w2029:dbl)
                        n4522 = local read "Position X"() -> (w2019:dbl)
                        n4523 = local read "Position Y"() -> (w2018:dbl)
                        n4524 = Number To Decimal String(number=w2017) -> (decimal integer string=w2014:string)  [unwired: 1 in]
                        n4525 = Number To Fractional String(number=w2035, precision (6)=i16 1) -> (F-format string=w2036:string)  [unwired: 2 in]
                        n4526 = Number To Fractional String(number=w2029, precision (6)=i16 1) -> (F-format string=w2031:string)  [unwired: 2 in]
                        n4527 = Number To Fractional String(number=w2019, precision (6)=i16 0) -> (F-format string=w2023:string)  [unwired: 2 in]
                        n4528 = Number To Fractional String(number=w2018, precision (6)=i16 0) -> (F-format string=w2027:string)  [unwired: 2 in]
                        n4529 = Concatenate Strings("Pixels de référence [X, Y] : [", w2036, ", ", w2031, "]") -> (w2021:string)
                        n4530 = Concatenate Strings("Position des tables [X, Y, Z] : ", w2023, ", ", w2027, "]") -> (w2020:string)
                        n4531 = Concatenate Strings("Lancement de l'asservissement (mode = '", w2014, "')") -> (w2013:string)
                        n4532 = Build Array(w2013, w2021, w2020) -> (w2038:string[])
                        n4533 = for {
                          tunnel: w2038 -> [w2039] mode=indexing
                          n4534 = control-ref of="TERMINAL"() -> (w2041:refnum<vi>)
                          n4535 = control-ref of="Indicateur d'état"() -> (w2040:refnum<vi>)
                          n4536 = call "TERMINAL.vi"("Indicateur Refnum"=w2040, "Terminal Refnum"=w2041, "Indicateur d'état"=w2039) -> ()
                        }
                      }
                    }
                  }
                  frame 4 {
                    w2042 = 0.0 ("GE_TCS_RA")
                    w2044 = T17."Disabled and Grayed Out" ("Disabled")
                    # "Mode de Guidage externe"
                    n4537 = local write "GE_TCS"(TRUE ("GE_TCS")) -> ()
                    n4538 = property on="StartServo" class="Bool (strict)"("DisabledEnum"=w2044) -> ()  [unwired: 2 in, 2 out]
                    n4539 = property on="Mode" class="MDér (strict)"("DisabledEnum"=w2044) -> ()  [unwired: 2 in, 2 out]
                    n4540 = local write "GE_TCS_DEC"(w2042) -> ()
                    n4541 = local write "GE_TCS_RA"(w2042) -> ()
                  }
                }
              }
              event "StopServo": Value Change {
                n4542 = event-data() -> ()  [unwired: 1 in, 5 out]
                n4543 = local read "Mode"() -> (w2045:u16)
                n4544 = case shown="0..3" w2045 {
                  frame 4 {
                    w2048 = T17."Enabled" ("Disabled")
                    n4545 = local write "GE_TCS"(FALSE ("GE_TCS")) -> ()
                    n4546 = property on="StartServo" class="Bool (strict)"("DisabledEnum"=w2048) -> ()  [unwired: 2 in, 2 out]
                    n4547 = property on="Mode" class="MDér (strict)"("DisabledEnum"=w2048) -> ()  [unwired: 2 in, 2 out]
                  }
                  frame Default {
                  }
                  frame 0..3 {
                    n4548 = flat-sequence {
                      frame #0 {
                        # "Quand le mode '0' est actif,\nPrAMS n'est pas au courant\net n'enverra l'événement \n\"emtTelescopeServoLevelChanged\""
                        n4549 = local read "Mode"() -> (w2049:u16)
                        n4550 = case shown="0" w2049 {
                          frame Default {
                          }
                          frame 0 {
                            n4551 = local write "Servo"(FALSE ("StopServo")) -> ()
                          }
                        }
                      }
                      frame #1 {
                        w2051 = u16 0 items=["Opération Fixe", "Asservissement Ouvert", "Asservissement Fermé", "Calibration"] ("Mode")
                        n4552 = control-ref of="PrAMS-ACK"() -> (w2056:refnum<vi>)
                        n4553 = local read "PrAMS VRN"() -> (w2059:refnum<visa-resource-name>)
                        n4554 = local read "PrAMS Error"() -> (w2058:errorcluster)
                        n4555 = local read "MessageType"() -> (w2055:cluster{string[], u32[]})
                        n4556 = control-ref of="PrAMS actif"() -> (w2057:refnum<vi>)
                        n4557 = local read "Signature"() -> (w2052:u32)
                        n4558 = call-poly "SAOMM-Num2littleEndian.vi"("Number"=w2051) -> ("LiitleEndianedData"=w2053:u8[])  [unwired: 14 in]
                        n4559 = call "SAOMM-SendSET.vi"("PRAMMS-COMM IN"=w2059, "Active Refnum"=w2057, "PrAMS-ACK"=w2056, "Signature"=w2052, "Error IN"=w2058, "MessageType"=w2055, "Active SET"="emtSetTelescopeServoLevel", "Value (little endianed byte array)"=w2053) -> ("PRAMMS-COMM OUT"=w2061:refnum<visa-resource-name>, "Error OUT"=w2060:errorcluster)  [unwired: 4 in, 2 out]
                        n4560 = local write "PrAMS Error"(w2060) -> ()
                        n4561 = local write "PrAMS VRN"(w2061) -> ()
                      }
                      frame #2 {
                        w2064 = TRUE
                        w2063 = T17."Enabled" ("Disabled")
                        n4562 = property on="StopCam" class="Bool (strict)"("DisabledEnum"=w2063) -> ()  [unwired: 2 in, 2 out]
                        n4563 = property on="StartServo" class="Bool (strict)"("DisabledEnum"=w2063) -> ()  [unwired: 2 in, 2 out]
                        n4564 = property on="XReference" class="NumNb (strict)"("DisabledEnum"=w2063) -> ()  [unwired: 2 in, 2 out]
                        n4565 = local write "Guidage en cour"(FALSE ("Guidage en cour")) -> ()
                        n4566 = local write "ForceSaveToFile"(w2064) -> ()
                        n4567 = local write "GuidingCancel"(w2064) -> ()
                        n4568 = property on="GoCam" class="Bool (strict)"("DisabledEnum"=w2063) -> ()  [unwired: 2 in, 2 out]
                        n4569 = property on="YReference" class="NumNb (strict)"("DisabledEnum"=w2063) -> ()  [unwired: 2 in, 2 out]
                        n4570 = property on="Mode" class="MDér (strict)"("DisabledEnum"=w2063) -> ()  [unwired: 2 in, 2 out]
                        n4571 = property on="Milieu" class="Bool (strict)"("DisabledEnum"=w2063) -> ()  [unwired: 2 in, 2 out]
                        n4572 = property on="exptime" class="NumNb (strict)"("DisabledEnum"=w2063) -> ()  [unwired: 2 in, 2 out]
                        n4573 = property on="AutoCentroid" class="Bool (strict)"("DisabledEnum"=w2063) -> ()  [unwired: 2 in, 2 out]
                        n4574 = property on="GetOptimal" class="Bool (strict)"("DisabledEnum"=w2063) -> ()  [unwired: 2 in, 2 out]
                      }
                      frame #3 {
                        w2066 = inf
                        n4575 = case shown="Vrai" TRUE {
                          frame False {
                          }
                          frame True {
                            w2079 = u16 2 items=["Opération Fixe", "Asservissement Ouvert", "Asservissement Fermé", "Calibration"] ("Mode")
                            n4576 = local write "Mode"(w2079) -> ()
                          }
                        }
                        n4577 = Initialize Array(0.0, 0) -> (w2076:dbl[])
                        n4578 = control-ref of="TCS actif"() -> (w2071:refnum<vi>)
                        n4579 = local read "TCS VRN"() -> (w2068:refnum<visa-resource-name>)
                        n4580 = Bundle(w2076, w2076) -> (w2074:cluster{dbl[], dbl[]})  [unwired: 1 in]
                        n4581 = Build Array(1.0 ("element")) -> (w2069:dbl[])
                        n4582 = Initialize Array(w2074, 0) -> (w2073:cluster{dbl[], dbl[]}[])
                        n4583 = local write "DiffX"(w2066) -> ()
                        n4584 = call "EXCOM-CMD.vi"("VRN IN"=w2068, "Bool Refnum"=w2071, "Commande #"=15, "Args"=w2069) -> ("VRN OUT"=w2067:refnum<visa-resource-name>)  [unwired: 9 in, 2 out]
                        n4585 = local write "Graph-Flux"(w2073) -> ()
                        n4586 = local write "Graph-Centroids"(w2073) -> ()
                        n4587 = local write "Graph-SNR"(w2073) -> ()
                        n4588 = local write "TCS VRN"(w2067) -> ()
                        n4589 = local write "DiffY"(w2066) -> ()
                        n4590 = local write "Hex-XGraph"(w2073) -> ()
                        n4591 = local write "Hex-YGraph"(w2073) -> ()
                        n4592 = local write "Guiderreur"(w2073) -> ()
                        n4593 = local write "Cumulatif"(w2073) -> ()
                      }
                    }
                  }
                }
                n4594 = local write "StopServo"(FALSE ("StopServo")) -> ()
              }
              event "SendHexOffset": Value Change {
                n4595 = event-data() -> ()  [unwired: 1 in, 5 out]
                n4596 = local write "SendHexOffset"(FALSE ("SendHexOffset")) -> ()
                n4597 = local read "MessageType"() -> (w2105:cluster{string[], u32[]})
                n4598 = control-ref of="Hexapod-ACK"() -> (w2111:refnum<vi>)
                n4599 = local read "Hexapod VRN"() -> (w2112:refnum<visa-resource-name>)
                n4600 = control-ref of="HexaCons actif"() -> (w2113:refnum<vi>)
                n4601 = local read "PrAMS Error"() -> (w2114:errorcluster)
                n4602 = call-poly "SAOMM-Num2littleEndian.vi"("Number"="Offset X") -> ("LiitleEndianedData"=w2097:u8[])  [unwired: 14 in]
                n4603 = call-poly "SAOMM-Num2littleEndian.vi"("Number"="Offset Y") -> ("LiitleEndianedData"=w2092:u8[])  [unwired: 14 in]
                n4604 = call-poly "SAOMM-Num2littleEndian.vi"("Number"="Offset Z") -> ("LiitleEndianedData"=w2091:u8[])  [unwired: 14 in]
                n4605 = call-poly "SAOMM-Num2littleEndian.vi"("Number"="Offset U") -> ("LiitleEndianedData"=w2088:u8[])  [unwired: 14 in]
                n4606 = call-poly "SAOMM-Num2littleEndian.vi"("Number"="Offset V") -> ("LiitleEndianedData"=w2087:u8[])  [unwired: 14 in]
                n4607 = local read "Signature"() -> (w2108:u32)
                n4608 = call "SAOMM-SendSET.vi"("PRAMMS-COMM IN"=w2112, "Active Refnum"=w2113, "PrAMS-ACK"=w2111, "Signature"=w2108, "Error IN"=w2114, "MessageType"=w2105, "Active SET"="emtSetXAxisOffset", "Value (little endianed byte array)"=w2097) -> ("PRAMMS-COMM OUT"=w2110:refnum<visa-resource-name>, "Error OUT"=w2101:errorcluster)  [unwired: 4 in, 2 out]
                n4609 = call "SAOMM-SendSET.vi"("PRAMMS-COMM IN"=w2110, "Active Refnum"=w2113, "PrAMS-ACK"=w2111, "Signature"=w2108, "Error IN"=w2101, "MessageType"=w2105, "Active SET"="emtSetYAxisOffset", "Value (little endianed byte array)"=w2092) -> ("PRAMMS-COMM OUT"=w2109:refnum<visa-resource-name>, "Error OUT"=w2102:errorcluster)  [unwired: 4 in, 2 out]
                n4610 = call "SAOMM-SendSET.vi"("PRAMMS-COMM IN"=w2109, "Active Refnum"=w2113, "PrAMS-ACK"=w2111, "Signature"=w2108, "Error IN"=w2102, "MessageType"=w2105, "Active SET"="emtSetZAxisOffset", "Value (little endianed byte array)"=w2091) -> ("PRAMMS-COMM OUT"=w2081:refnum<visa-resource-name>, "Error OUT"=w2103:errorcluster)  [unwired: 4 in, 2 out]
                n4611 = call "SAOMM-SendSET.vi"("PRAMMS-COMM IN"=w2081, "Active Refnum"=w2113, "PrAMS-ACK"=w2111, "Signature"=w2108, "Error IN"=w2103, "MessageType"=w2105, "Active SET"="emtSetUAxisOffset", "Value (little endianed byte array)"=w2088) -> ("PRAMMS-COMM OUT"=w2080:refnum<visa-resource-name>, "Error OUT"=w2104:errorcluster)  [unwired: 4 in, 2 out]
                n4612 = call "SAOMM-SendSET.vi"("PRAMMS-COMM IN"=w2080, "Active Refnum"=w2113, "PrAMS-ACK"=w2111, "Signature"=w2108, "Error IN"=w2104, "MessageType"=w2105, "Active SET"="emtSetVAxisOffset", "Value (little endianed byte array)"=w2087) -> ("PRAMMS-COMM OUT"=w2082:refnum<visa-resource-name>, "Error OUT"=w2083:errorcluster)  [unwired: 4 in, 2 out]
                n4613 = case shown="Pas d'erreur" w2083 {
                  selector: w2083 -> [w2117 w2126]
                  tunnel: w2113 -> [w2125 _]
                  tunnel: w2111 -> [w2124 _]
                  tunnel: w2108 -> [w2123 _]
                  tunnel: [w2122 w2127] -> w2107
                  tunnel: [w2121 w2126] -> w2106
                  tunnel: w2105 -> [w2120 _]
                  tunnel: "emtApplyAxesOffsets" -> [w2119 _]
                  tunnel: u8[] [] ("Value (little endianed byte array)") -> [w2118 _]
                  tunnel: w2082 -> [w2116 w2127]
                  frame No Error {
                    n4614 = call "SAOMM-SendSET.vi"("PRAMMS-COMM IN"=w2116, "Active Refnum"=w2125, "PrAMS-ACK"=w2124, "Signature"=w2123, "Error IN"=w2117, "MessageType"=w2120, "Active SET"=w2119, "Value (little endianed byte array)"=w2118) -> ("PRAMMS-COMM OUT"=w2122:refnum<visa-resource-name>, "Error OUT"=w2121:errorcluster)  [unwired: 4 in, 2 out]
                  }
                  frame Error {
                  }
                }
                n4615 = local write "Hexapod VRN"(w2107) -> ()
                n4616 = local write "PrAMS Error"(w2106) -> ()
              }
              event "HexRAZ": Value Change {
                n4617 = event-data() -> ()  [unwired: 1 in, 5 out]
                n4618 = local read "Signature"() -> (w2135:u32)
                n4619 = control-ref of="Hexapod-ACK"() -> (w2137:refnum<vi>)
                n4620 = local read "Hexapod VRN"() -> (w2136:refnum<visa-resource-name>)
                n4621 = local read "PrAMS Error"() -> (w2134:errorcluster)
                n4622 = local read "MessageType"() -> (w2133:cluster{string[], u32[]})
                n4623 = control-ref of="HexaCons actif"() -> (w2138:refnum<vi>)
                n4624 = local read "HexU"() -> (w2132:dbl)
                n4625 = local read "HexV"() -> (w2131:dbl)
                n4626 = local write "HexRAZ"(FALSE ("HexRAZ")) -> ()
                n4627 = call "SAOMM-RaZ.vi"("PRAMMS-COMM IN"=w2136, "Active Refnum"=w2138, "PrAMS-ACK"=w2137, "Signature"=w2135, "Error IN"=w2134, "MessageType"=w2133, "Position U"=w2132, "Position V"=w2131) -> ("PRAMMS-COMM OUT"=w2130:refnum<visa-resource-name>, "Error OUT"=w2129:errorcluster)  [unwired: 6 in]
                n4628 = local write "Hexapod VRN"(w2130) -> ()
                n4629 = local write "PrAMS Error"(w2129) -> ()
              }
            }
            n4630 = local read "Quit"() -> (w1440:bool)
          }
          "PrAMS + SAOMM" <- w975
          n4631 = while {
            shift-right: [w2150] -> _
            shift-left: w985 -> [w2149]
            tunnel: w984 -> [w2145]
            tunnel: [w2143] -> w974
            i -> [w2139]
            stop <- w2143 stop-if-true
            # "ms to wait for 1st 4 bytes"
            n4632 = local read "MessageType"() -> (w2152:cluster{string[], u32[]})
            n4633 = local read "Signature"() -> (w2144:u32)
            n4634 = local read "PrAMS VRN"() -> (w2155:refnum<visa-resource-name>)
            n4635 = local read "PrAMS Error"() -> (w2154:errorcluster)
